vi "Convert Image to Binary U8s.vi"(10 "Image Dst":T1, 11 "ImageIn":T1) -> (1 "Timimngs":u32[](array[numeric]), 3 "Image Out":T1)   [LabVIEW 2015]
uses:
  <vilib>/vision/Image Controls.llb/IMAQ Image.ctl
  <vilib>/vision/NI_Vision_Development_Module.lvlib
panel:
  in  "Color Plane":i32(ring) items=["Red", "Green", "Blue", "Hue", "Saturation", "Luminance", "Value", "Intensity"]
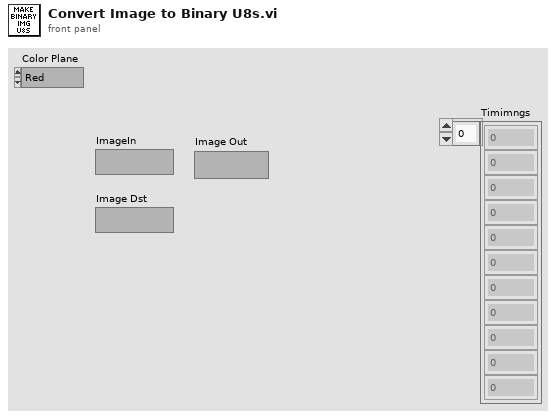
[diagram p1: front panel]
types:
  T1 = typedef "IMAQ Image.ctl" = refnum<image>
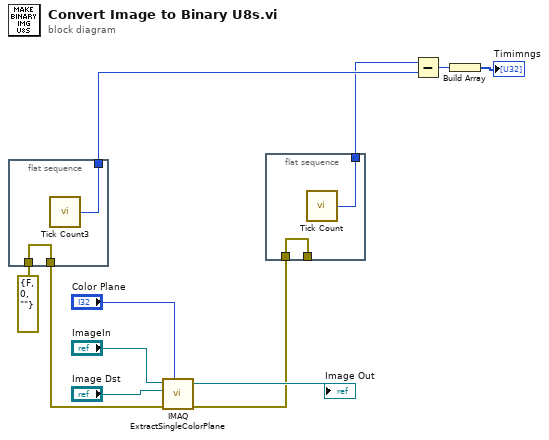
[diagram p0: block diagram]
diagram:
  n1 = flat-sequence {
    tunnel: errorcluster {"status"=FALSE, "code"=0, "source"=""} ("error out") -> [w13]
    tunnel: [w13] -> w8
    tunnel: [w12] -> w6
    frame #0 {
      n2 = call "Tick Count3"() -> ("Tick Count(mSec)"=w12:u32)
    }
  }
  n3 = call "IMAQ ExtractSingleColorPlane"("Color Plane"="Color Plane", "error in (no error)"=w8, "Image Dst"="Image Dst", "Image Src"="ImageIn") -> ("error out"=w2:errorcluster, "Image Dst Out"=→"Image Out":T1)  [unwired: 6 out]
  n4 = flat-sequence {
    tunnel: w2 -> [w15]
    tunnel: [w15] -> _
    tunnel: [w14] -> w1
    frame #0 {
      n5 = call "Tick Count"() -> ("Tick Count(mSec)"=w14:u32)
    }
  }
  n6 = Subtract(x=w1, y=w6) -> (x-y=w5:u32)
  n7 = Build Array(w5) -> (→"Timimngs":u32[])
